vi "Get Flow Rate Setpoint.vi"(8 "error in (no error)":errorcluster, 11 "RRG in":refnum<class "PL Eltochpribor RRG.lvclass">) -> (0 "error out":errorcluster, 2 "flow rate setpoint, %":dbl, 3 "RRG out":refnum<class "PL Eltochpribor RRG.lvclass">)   [LabVIEW 2015, in "PL Eltochpribor RRG.lvclass"]
doc: "Gets flow rate setpoint as a percentage of full scale calibrated flow rate."
uses:
  PL Eltochpribor RRG.lvclass
  <vilib>/plasmapper/PL Modbus Client/PL Modbus Client.lvclass
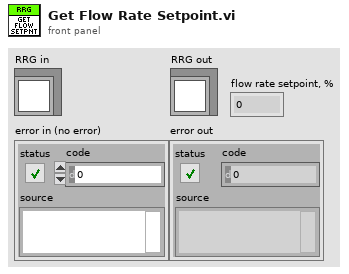
[diagram p1: front panel]
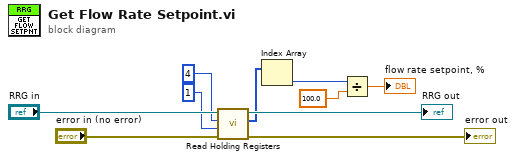
[diagram p0: block diagram]
diagram:
  n1 = call <vilib>:"Read Holding Registers.vi"("error in (no error)"="error in (no error)", "number of holding registers"=u16 1, "address"=u16 4, "MODBUS in"="RRG in") -> ("error out"=→"error out":errorcluster, "values"=w4:u16[], "MODBUS out"=→"RRG out":refnum<class "PL Eltochpribor RRG.lvclass">)  [unwired: 5 in]
  n2 = Index Array(array=w4) -> (element=w1:u16)  [unwired: 1 in]
  n3 = Divide(x=w1, y=100.0) -> (x/y=→"flow rate setpoint, %":dbl)
